vi "Dot Product PtByPt.vi"(2 "initialize":bool, 3 "sample length":i32=100, 4 "x":dbl format="%0.2f", 5 "y":dbl format="%0.2f") -> (0 "error":i32, 1 "X*Y":dbl format="%0.2f")   [LabVIEW 2020, in "NI_PtbyPt.lvlib"]
doc: "Computes the dot product, <B>X*Y</B>, of <B>y</B> and <B>x</B>."
uses:
  NI_PtbyPt.lvlib
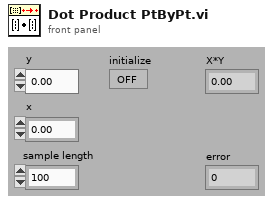
[diagram p1: front panel]
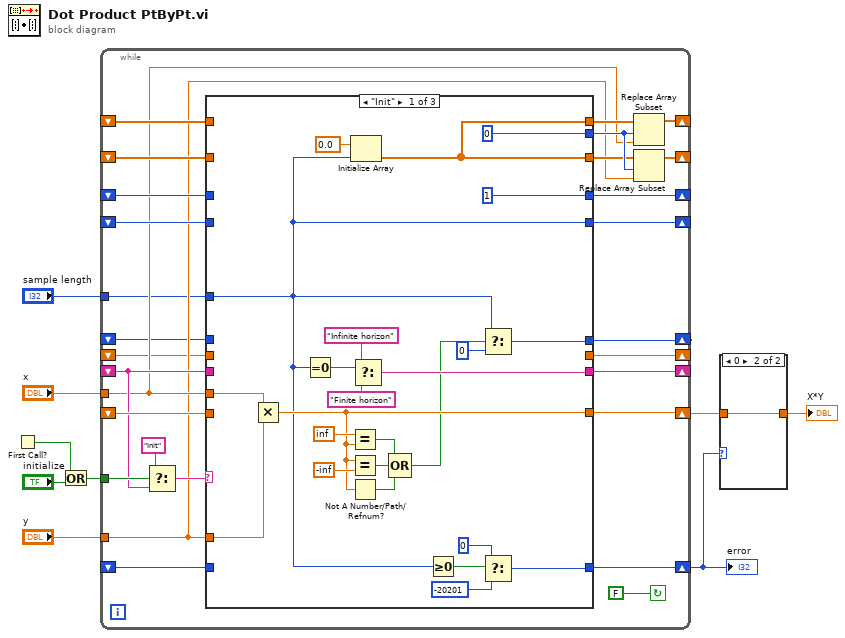
[diagram p0: block diagram]
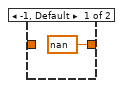
[diagram p2: hidden frame]
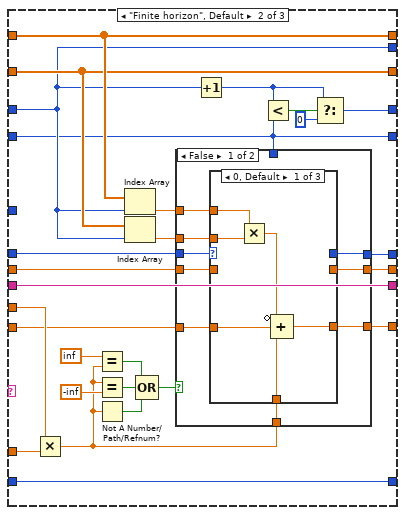
[diagram p3: hidden frame]
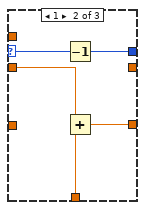
[diagram p4: hidden frame]
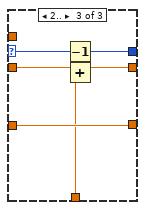
[diagram p5: hidden frame]
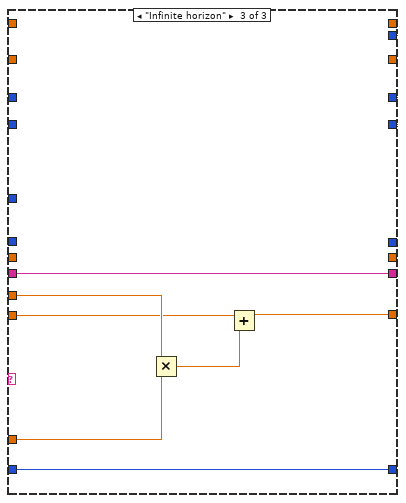
[diagram p7: hidden frame]
diagram:
  n1 = First Call?() -> (First Call?: T/F=w6:bool)
  n2 = Or(x=w6, y="initialize") -> (x .or. y?=w7:bool)
  n3 = while {
    tunnel: w7 -> [w25]
    shift-left: _ -> [w23]
    shift-right: [w21] -> _
    shift-left: _ -> [w26]
    shift-right: [w27] -> _
    shift-left: _ -> [w28]
    shift-right: [w29] -> w2
    shift-left: _ -> [w31]
    shift-right: [w17] -> _
    shift-left: _ -> [w30]
    shift-right: [w36] -> _
    shift-left: _ -> [w34]
    shift-right: [w37] -> _
    tunnel: "x" -> [w19]
    tunnel: "y" -> [w18]
    shift-right: [w16] -> _
    shift-left: _ -> [w15]
    shift-right: [w14] -> _
    shift-left: _ -> [w13]
    tunnel: "sample length" -> [w12]
    shift-right: [w11] -> w3
    shift-left: _ -> [w10]
    stop <- FALSE continue-if-true
    n4 = Select(t="Init", s=w25, f=w23) -> (s? t:f=w22:string)
    n5 = case shown="\"Init\"" w22 {
      tunnel: w18 -> [w60 w88 w122]
      tunnel: w19 -> [w61 w87 w123]
      tunnel: [1 w65 w119] -> w17
      tunnel: [0 ("Index") w66 w119] -> w35
      tunnel: w26 -> [_ w63 _]
      tunnel: w34 -> [_ w85 _]
      tunnel: [w56 w85 _] -> w33
      tunnel: [w56 w84 _] -> w32
      tunnel: w31 -> [_ w66 _]
      tunnel: w30 -> [_ w84 _]
      tunnel: [w42 w82 w120] -> w29
      tunnel: w28 -> [_ w81 w121]
      tunnel: [w41 w63 w119] -> w27
      tunnel: [w52 w80 w118] -> w21
      tunnel: w23 -> [_ w80 w118]
      tunnel: [w40 w72 _] -> w16
      tunnel: w15 -> [_ w71 _]
      tunnel: [_ w70 _] -> w14
      tunnel: w13 -> [_ w69 _]
      tunnel: w12 -> [w41 _ _]
      tunnel: [w48 w62 w117] -> w11
      tunnel: w10 -> [_ w62 w117]
      frame "Init" {
        n6 = Multiply(x=w61, y=w60) -> (x*y=w42:dbl)
        n7 = Equal To 0?(x=w41) -> (x = 0?=w55:bool)
        n8 = Equal?(x=inf, y=w42) -> (x = y?=w44:bool)
        n9 = Equal?(x=w42, y=-inf) -> (x = y?=w45:bool)
        n10 = Not A Number/Path/Refnum?(number/path/refnum=w42) -> (NaN/Path/Refnum?=w43:bool)
        n11 = Initialize Array(0.0 ("Element Data"), w41) -> (w56:dbl[])
        n12 = Select(t="Infinite horizon", s=w55, f="Finite horizon") -> (s? t:f=w52:string)
        n13 = Compound Arithmetic op=OR(w44, w45, w43) -> (w39:bool)
        n14 = Greater Or Equal To 0?(x=w41) -> (x >= 0?=w51:bool)
        n15 = Select(t=w41, s=w39, f=0) -> (s? t:f=w40:i32)
        n16 = Select(t=0, s=w51, f=-20201) -> (s? t:f=w48:i32)
      }
      frame "Finite horizon", Default {
        n17 = Multiply(x=w87, y=w88) -> (x*y=w74:dbl)
        n18 = Equal?(x=inf, y=w74) -> (x = y?=w76:bool)
        n19 = Equal?(x=w74, y=-inf) -> (x = y?=w77:bool)
        n20 = Not A Number/Path/Refnum?(number/path/refnum=w74) -> (NaN/Path/Refnum?=w75:bool)
        n21 = Index Array(array=w85, index=w66) -> (element=w86:dbl)
        n22 = Index Array(array=w84, index=w66) -> (element=w83:dbl)
        n23 = Compound Arithmetic op=OR(w76, w77, w75) -> (w73:bool)
        n24 = case shown="False" w73 {
          tunnel: w86 -> [w97 _]
          tunnel: w83 -> [w96 _]
          tunnel: [w95 w116] -> w82
          tunnel: w81 -> [w94 _]
          tunnel: w74 -> [w93 w116]
          tunnel: [w89 w115] -> w72
          tunnel: w71 -> [w92 _]
          tunnel: [w91 _] -> w70
          tunnel: w69 -> [w90 _]
          tunnel: w63 -> [_ w115]
          frame False {
            n25 = case shown="0, Default" w92 {
              selector: w92 -> [_ w105 w110]
              tunnel: w97 -> [w103 _ _]
              tunnel: w96 -> [w102 _ _]
              tunnel: [w101 w108 w114] -> w95
              tunnel: w94 -> [w100 _ w114]
              tunnel: w93 -> [w99 w107 w112]
              tunnel: [_ _ w113] -> w91
              tunnel: w90 -> [_ w106 w111]
              tunnel: [_ w104 w109] -> w89
              frame 0, Default {
                n26 = Multiply(x=w103, y=w102) -> (x*y=w98:dbl)
                n27 = Compound Arithmetic op=ADD(invert w98, w100, w99) -> (w101:dbl)
              }
              frame 1 {
                n28 = Decrement(x=w105) -> (x-1=w104:i32)
                n29 = Add(x=w106, y=w107) -> (x+y=w108:dbl)
              }
              frame 2.. {
                n30 = Decrement(x=w110) -> (x-1=w109:i32)
                n31 = Add(x=w111, y=w112) -> (x+y=w113:dbl)
              }
            }
          }
          frame True {
          }
        }
        n32 = Increment(x=w66) -> (x+1=w64:i32)
        n33 = Less?(x=w64, y=w63) -> (x < y?=w67:bool)
        n34 = Select(t=w64, s=w67, f=0 ("Index")) -> (s? t:f=w65:i32)
      }
      frame "Infinite horizon" {
        w119 = 0 ("Index")
        n35 = Multiply(x=w123, y=w122) -> (x*y=w124:dbl)
        n36 = Add(x=w121, y=w124) -> (x+y=w120:dbl)
      }
    }
    n37 = Replace Array Subset(array=w33, new element=w19, index=w35) -> (w37:dbl[])
    n38 = Replace Array Subset(array=w32, new element=w18, index=w35) -> (w36:dbl[])
  }
  "error" <- w3
  n39 = case shown="0" w3 {
    tunnel: w2 -> [_ w126]
    tunnel: [nan w126] -> w1
    frame -1, Default {
    }
    frame 0 {
    }
  }
  "X*Y" <- w1
